vi "Get_measurement_samplingdata.vi"(0 "SPU":refnum<k24>, 1 "STSProcess.ILSTS":refnum<k24>, 2 "TSL":refnum<k24>, 5 "Meas_monitor_struct":refnum<k24>[](array[refnum]), 7 "MPM":refnum<k24>[](array[refnum]), 9 "Data_struct":refnum<k24>[](array[refnum]), 11 "错误输入（无错误）":errorcluster, 12 "SweepCount":i32) -> (15 "error out":errorcluster)   [LabVIEW 2017]
doc: "Get logging measurement data & add in"
uses:
  D:/test/ILSTS/LV_IL/LV_IL_Sample_x64/DLL/STSProcess.dll
  DLL/STSProcess.dll
  D:/test/ILSTS/LV_IL/LV_IL_Sample_x64/DLL/InstrumentDLL.dll
  DLL/InstrumentDLL.dll
  Share/PowerMonitorType.vi
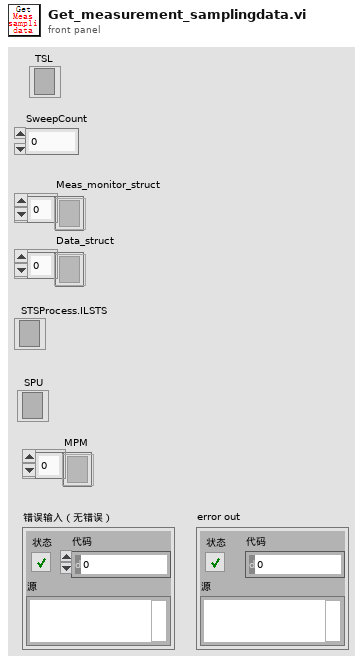
[diagram p1: front panel]
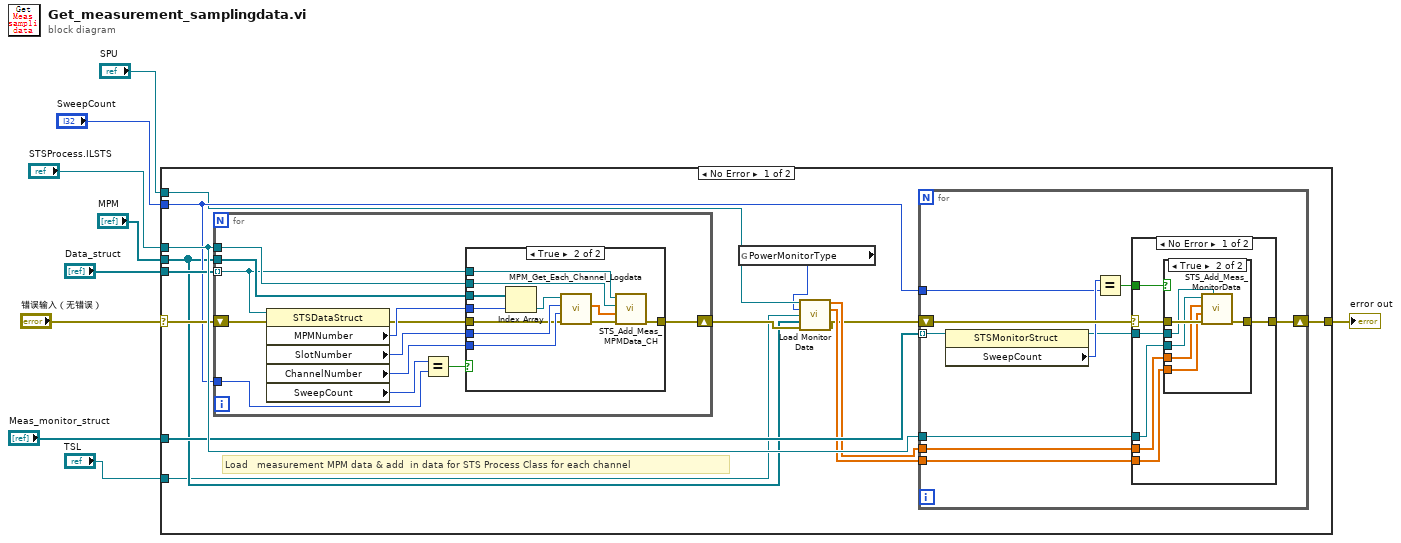
[diagram p0: block diagram]
diagram:
  n1 = case shown="No Error" "错误输入（无错误）" {
    selector: "错误输入（无错误）" -> [w19 w73]
    tunnel: "STSProcess.ILSTS" -> [w23 _]
    tunnel: "Meas_monitor_struct" -> [w22 _]
    tunnel: "SPU" -> [w14 _]
    tunnel: "MPM" -> [w12 _]
    tunnel: "Data_struct" -> [w21 _]
    tunnel: [w20 w73] -> w6
    tunnel: "SweepCount" -> [w18 _]
    tunnel: "TSL" -> [w11 _]
    frame No Error {
      # "Load　measurement MPM data & add  in data for STS Process Class for each channel"
      n2 = for {
        tunnel: w21 -> [w52] mode=indexing
        tunnel: w12 -> [w58]
        tunnel: w23 -> [w53]
        tunnel: w18 -> [w50]
        shift-right: [w54] -> w13
        shift-left: w19 -> [w55]
        n3 = property on="属性节点" class="STSDataStruct"(reference=w52, error in=w55) -> (error out=w56:errorcluster, "MPMNumber"=w57:i32, "SlotNumber"=w60:i32, "ChannelNumber"=w59:i32, "SweepCount"=w51:i32)  [unwired: 1 out]
        n4 = Equal?(x=w51, y=w50) -> (x = y?=w49:bool)
        n5 = case shown="True" w49 {
          tunnel: w60 -> [_ w72]
          tunnel: w59 -> [_ w71]
          tunnel: w58 -> [_ w70]
          tunnel: w57 -> [_ w69]
          tunnel: w56 -> [w61 w68]
          tunnel: [w61 w66] -> w54
          tunnel: w53 -> [_ w63]
          tunnel: w52 -> [_ w62]
          frame False {
          }
          frame True {
            n6 = Index Array(array=w70, index=w69) -> (element=w67:refnum<k24>)
            n7 = call "MPM_Get_Each_Channel_Logdata.vi"("error in (no error)"=w68, "channelNumber"=w71, "moduleNumber"=w72, ".NET Reference in"=w67) -> ("error out"=w65:errorcluster, "data out"=w64:sgl[])  [unwired: 5 in, 1 out]
            n8 = call "STS_Add_Meas_MPMData_CH.vi"("错误输入（无错误）"=w65, "data"=w64, "STSProcess.ILSTS"=w63, ".NET引用句柄输入"=w62) -> ("错误输出"=w66:errorcluster)  [unwired: 6 in, 1 out]
          }
        }
      }
      n9 = global read "PowerMonitorType.vi" "PowerMonitorType"() -> (w10:enum16{"DAQ", "MPM_220", "TSL_LOGG"})
      n10 = call "Load Monitor Data.vi"("SPU"=w14, "PowerMonitorType"=w10, "TSL"=w11, "MPM"=w12, "error in (no error)"=w13) -> ("trigger"=w17:sgl[], "monitor"=w16:sgl[], "error out"=w15:errorcluster)  [unwired: 8 in]
      n11 = for {
        tunnel: w22 -> [w28] mode=indexing
        tunnel: w23 -> [w33]
        tunnel: w17 -> [w32]
        tunnel: w16 -> [w31]
        shift-right: [w29] -> w20
        shift-left: w15 -> [w30]
        tunnel: w18 -> [w26]
        n12 = property on="属性节点" class="STSMonitorStruct"(reference=w28) -> (reference out=w24:refnum<k24>, "SweepCount"=w27:i32)  [unwired: 1 in, 1 out]
        n13 = Equal?(x=w27, y=w26) -> (x = y?=w25:bool)
        n14 = case shown="No Error" w30 {
          selector: w30 -> [w39 w48]
          tunnel: w33 -> [w38 _]
          tunnel: w24 -> [w35 _]
          tunnel: w32 -> [w37 _]
          tunnel: w31 -> [w36 _]
          tunnel: [w40 w48] -> w29
          tunnel: w25 -> [w34 _]
          frame No Error {
            n15 = case shown="True" w34 {
              tunnel: [w41 w47] -> w40
              tunnel: w39 -> [w41 w46]
              tunnel: w38 -> [_ w45]
              tunnel: w37 -> [_ w44]
              tunnel: w36 -> [_ w43]
              tunnel: w35 -> [_ w42]
              frame False {
              }
              frame True {
                n16 = call "STS_Add_Meas_MonitorData.vi"("setting"=w42, "错误输入（无错误）"=w46, "monitorData"=w43, "triggerIndex"=w44, "STSProcess.ILSTS"=w45) -> ("错误输出"=w47:errorcluster)  [unwired: 5 in, 1 out]
              }
            }
          }
          frame Error {
          }
        }
      }
    }
    frame Error {
    }
  }
  "error out" <- w6
